vi "Log Clear.vi"(8 "error in (no error)":errorcluster caption="エラー入力 (エラーなし)" {"code" format="%.0x"}, 11 "Result Log Reference":refnum<vi>) -> (0 "error out":errorcluster caption="エラー出力" {"code" format="%.0x"}, 3 "Result Log Reference Out":refnum<vi>)   [LabVIEW 2020]
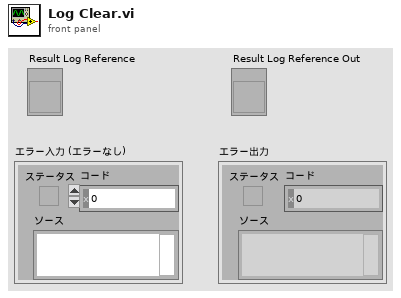
[diagram p1: front panel]
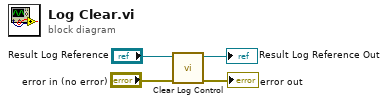
[diagram p0: block diagram]
diagram:
  n1 = call "Clear Log Control.vi"("エラー入力 (エラーなし)"="error in (no error)", "Result Log Reference"="Result Log Reference") -> ("エラー出力"=→"error out":errorcluster, "Result Log Reference Out"=→"Result Log Reference Out":refnum<vi>)  [unwired: 8 in]
